vi "tb_SPI API (Host).vi"() -> ()   [LabVIEW 2014]
doc: "This example shows simulation of SPI API on Host Computer. This is used to quickly check the correctness of settings to communicate with SPI Slave in software before proceeding to actual hardware."
uses:
  user.lib/_NI SPI IP/FPGA/Controllers/Public/Spi Master Inputs.ctl
  user.lib/_NI SPI IP/FPGA/Controllers/Public/Transfer Settings.ctl
  Controls/SPI Response Information.ctl
panel:
  out "SPI Response Data":T1
  in  "Stop":bool
  out "Digital Data":digitalwaveform(graph)
  in  "SPI PHY Settings":T2={"Divide Value"=20, "Transfer Length (bits)"=8, "CS Asserted Polarity"=FALSE, "Clock Polarity (CPOL)"=FALSE, "Clock Phase (CPHA)"=FALSE, "Lengthen MISO Setup"=FALSE, "Direction Change Bit"=0, "MOSI Starts as Output"=FALSE, "Tristatable MOSI"=FALSE} {"Direction Change Bit" max=64 step=1; "Transfer Length (bits)" min=1 max=64 step=1}
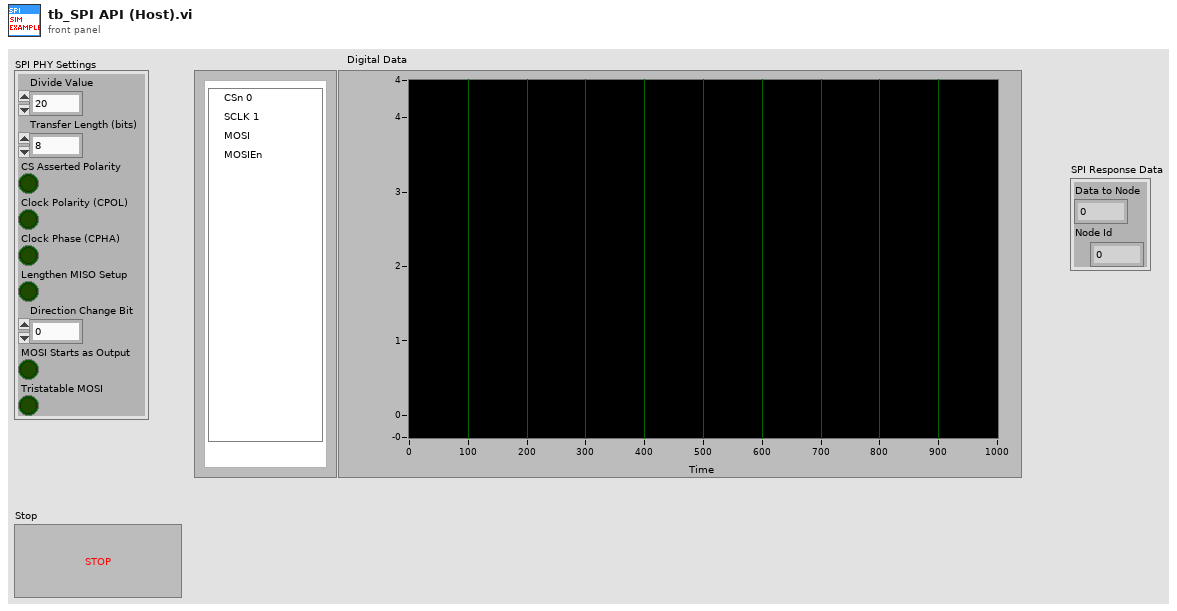
[diagram p1: front panel]
types:
  T1 = typedef "SPI Response Information.ctl" = cluster{"Data to Node":u64, "Node Id":u16}
  T2 = typedef "NI SPI IP (FPGA).lvlib/Transfer Settings.ctl" = cluster{"Divide Value":u8, "Transfer Length (bits)":u8, "CS Asserted Polarity":bool, "Clock Polarity (CPOL)":bool, "Clock Phase (CPHA)":bool, "Lengthen MISO Setup":bool, "Direction Change Bit":u8, "MOSI Starts as Output":bool, "Tristatable MOSI":bool}
  T3 = typedef "Internal Data (SPI API).ctl" = cluster{"DLU To SPI Engine Data FIFO":refnum<k21>, "SPI Engine to DLU Data FIFO":refnum<k21>, "Data to SPI Engine (Cache) Register":refnum<k21>, "SPI PHY Settings to SPI Engine (Cahche) Register":refnum<k21>}
  T4 = typedef "NI SPI IP (FPGA).lvlib/Spi Master Inputs.ctl" = cluster{"MISO":bool}
  T5 = typedef "NI SPI IP FPGA.lvlib/Spi Master Outputs.ctl" = cluster{"Chip Select":bool, "Clock":bool, "MOSI":bool, "MOSI OE":bool}
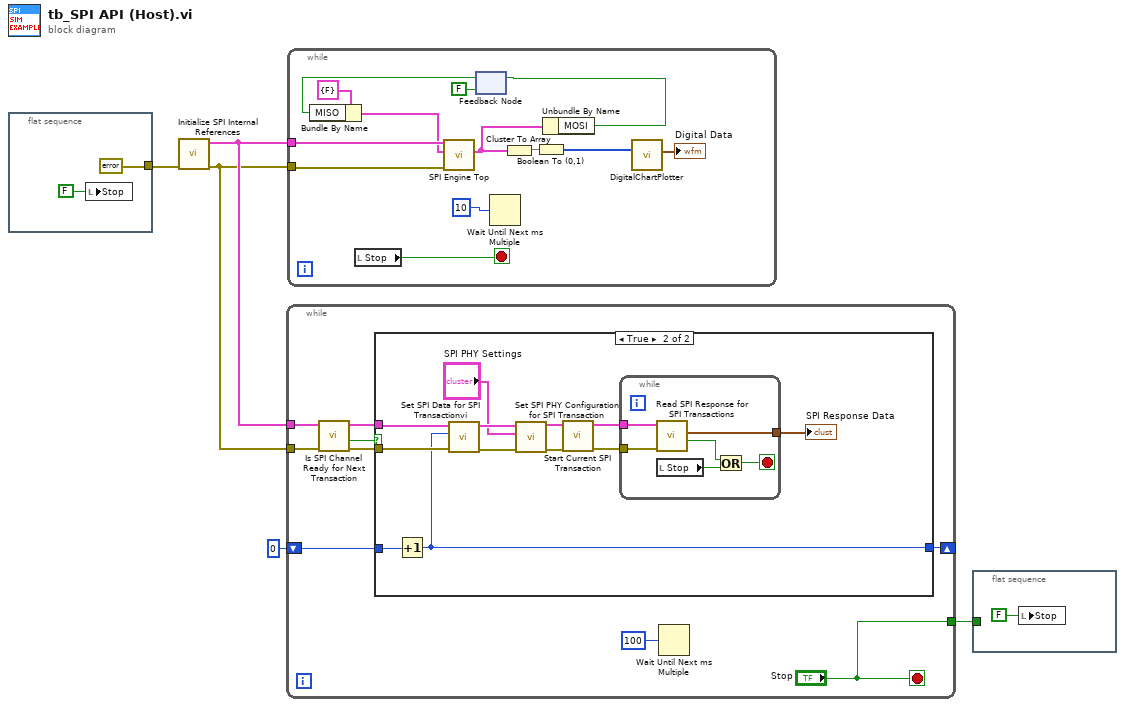
[diagram p0: block diagram]
diagram:
  n1 = flat-sequence {
    tunnel: [errorcluster {"status"=FALSE, "code"=0, "source"=""} ("error in")] -> w2
    frame #0 {
      n2 = local write "Stop"(FALSE ("Stop")) -> ()
    }
  }
  n3 = call "Initialize SPI Internal References.vi"("error in"=w2) -> ("error out"=w4:errorcluster, "SPI API References"=w5:T3)  [unwired: 9 in]
  n4 = while {
    tunnel: w5 -> [w16]
    tunnel: w4 -> [w15]
    shift-right: [w10] -> _
    shift-left: u8 0 -> [w11]
    tunnel: ["Stop"] -> w1
    stop <- "Stop" stop-if-true
    n5 = call "Is SPI Channel Ready for Next Transaction.vi"("error in"=w15, "Private Data In"=w16) -> ("error out"=w12:errorcluster, "SPI Channel Ready"=w14:bool, "Private Data Out"=w13:T3)  [unwired: 6 in, 1 out]
    n6 = case shown="True" w14 {
      tunnel: w13 -> [_ w29]
      tunnel: w12 -> [_ w28]
      tunnel: w11 -> [w17 w21]
      tunnel: [w17 w19] -> w10
      frame False {
      }
      frame True {
        n7 = Increment(x=w21) -> (x+1=w19:u8)
        n8 = call "Set SPI Data for SPI Transactionvi.vi"("error in"=w28, "Data In"=w19, "Private Data In"=w29) -> ("error out"=w26:errorcluster, "Private Data Out"=w27:T3)  [unwired: 7 in]
        n9 = call "Set SPI PHY Configuration for SPI Transaction.vi"("error in"=w26, "SPI PHY Settings"="SPI PHY Settings", "Private Data In"=w27) -> ("error out"=w24:errorcluster, "Private Data Out"=w25:T3)  [unwired: 7 in]
        n10 = call "Start Current SPI Transaction.vi"("error in"=w24, "Private Data In"=w25) -> ("error out"=w22:errorcluster, "Private Data Out"=w23:T3)  [unwired: 7 in, 1 out]
        n11 = while {
          tunnel: w23 -> [w35]
          tunnel: w22 -> [w34]
          tunnel: [w33] -> w18
          stop <- w30 stop-if-true
          n12 = call "Read SPI Response for SPI Transactions.vi"("error in"=w34, "Private Data In"=w35) -> ("Read Data Valid?"=w32:bool, "Read Data"=w33:T1)  [unwired: 6 in, 2 out]
          n13 = local read "Stop"() -> (w31:bool)
          n14 = Or(x=w32, y=w31) -> (x .or. y?=w30:bool)
        }
        "SPI Response Data" <- w18
      }
    }
    n15 = Wait Until Next ms Multiple(millisecond multiple=u32 100) -> ()  [unwired: 1 out]
  }
  n16 = while {
    tunnel: w5 -> [w48]
    tunnel: w4 -> [w47]
    stop <- w45 stop-if-true
    n17 = local read "Stop"() -> (w45:bool)
    n18 = feedback #1(FALSE ("MOSI")) -> (w41:bool)
    n19 = Bundle By Name(cluster=T4 {"MISO"=FALSE} ("SPI DIO Input"), "MISO"=w41) -> (w43:T4)
    n20 = call "SPI Engine Top.vi"("error in"=w47, "SPI Read Data"=w43, "SPI API References"=w48) -> ("SPI DIO Output"=w38:T5)  [unwired: 5 in, 3 out]
    n21 = Wait Until Next ms Multiple(millisecond multiple=u32 10) -> ()  [unwired: 1 out]
    n22 = Cluster To Array(cluster=w38) -> (array=w37:bool[])
    n23 = Boolean To (0,1)(Boolean=w37) -> (0, 1=w36:i16[])
    n24 = Unbundle By Name(w38) -> ("MOSI"=w42:bool)
    n25 = feedback-in #1(w42) -> ()
    n26 = call "DigitalChartPlotter.vi"("Input"=w36) -> ("Digital Data"=→"Digital Data":digitalwaveform)  [unwired: 10 in]
  }
  n27 = flat-sequence {
    tunnel: w1 -> [_]
    frame #0 {
      n28 = local write "Stop"(FALSE ("Stop")) -> ()
    }
  }
